vi "construct_shutdown.vi"(11 "error in (no error) 2":errorcluster) -> (4 "command out":T1=enum."configure_rf", 6 "parameters JSON":string, 10 "data out":variant, 14 "Debug info":string, 15 "error out 2":errorcluster)   [LabVIEW 2019, in "mmW_commands.lvlib"]
uses:
  mmW_commands.lvlib
  <vilib>/addons/_JKI.lib/Serialization/JSON/JKI JSON Serialization.lvlib
  TypeDefs/_depr_datatypes.ctl
  shutdown_typedef.ctl
  TypeDefs/commands.ctl
panel:
  out "datatype (only for debug)":T2
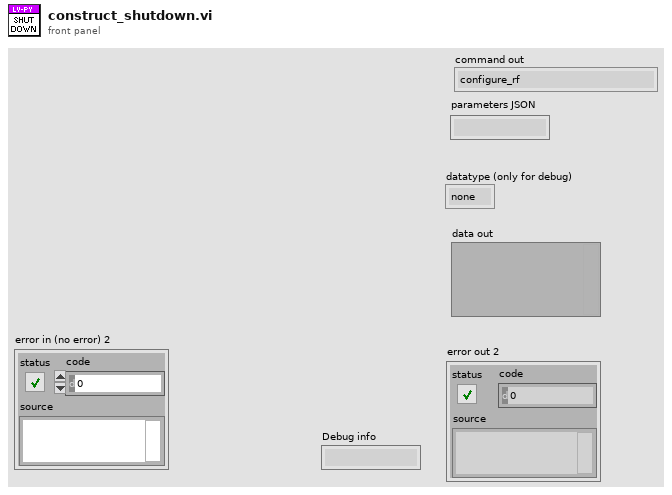
[diagram p1: front panel]
types:
  T1 = typedef "mmW_commands.lvlib/commands.ctl" = enum16{"configure_fs", "configure_rf", "configure_trigger", "equalization_enable", "equalization_start", "lo_sync_enable", "equalization_stop", "get_instrument_status", "get_versions", "initialize_hw", "pop_rx", "set_log_level", "Shutdown", "start", "start_instrument_app", "stop", "trans", "transceive", "trigger_burst", "trigger_sync_enable", "Write TX", "resp_generic", "resp_waveform", "send_trigger", "fetch", "transceive2"}
  T2 = typedef "mmW_commands.lvlib/_depr_datatypes.ctl" = enum16{"none", "float", "string", "CSG_wfm", "DBL_wfm"}
  T3 = typedef "mmW_commands.lvlib/shutdown_typedef.ctl" = cluster{"datatype":string}
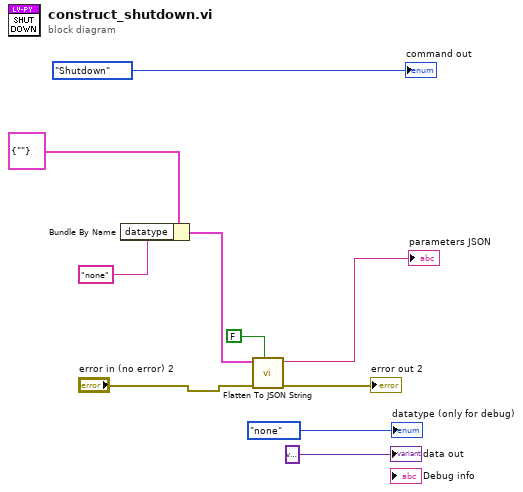
[diagram p0: block diagram]
diagram:
  n1 = Bundle By Name(cluster=T3 {"datatype"=""} ("Cluster"), "datatype"="none") -> (w9:T3)
  n2 = call <vilib>:"Flatten To JSON String.vi"("Multiline (T)"=FALSE, "error in (no error)"="error in (no error) 2", "Variant"=w9) -> ("error out"=→"error out 2":errorcluster, "JSON String"=→"parameters JSON":string)  [unwired: 7 in]
  "datatype (only for debug)" <- _depr_datatypes."none" ("datatypes")
  "data out" <- variant
  "command out" <- commands."Shutdown" ("mmW_instrument_commands")
